vi "Build descriptor.vi"(11 "Builder in":refnum<class "Builder.lvclass">) -> (3 "Builder out":refnum<class "Builder.lvclass">)   [LabVIEW 2025, in "App-Builder Library.lvlib" / "Builder.lvclass"]
uses:
  Builder.lvclass
  Builder.lvclass/Builder.ctl
  App descriptions.ctl
  Build Type.ctl
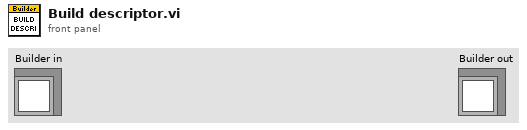
[diagram p1: front panel]
types:
  T1 = typedef "App-Builder Library.lvlib/Builder.lvclass/Build specification.ctl" = cluster{"target name":string, "Build specification":string, "Project Path":path, "Build Object type":T2}
  T2 = typedef "App-Builder Library.lvlib/Builder.lvclass/Build object type.ctl" = enum16{"EXE", "RT EXE", "Deployable Packed"}
  T3 = typedef "App-Builder Library.lvlib/Builder.lvclass/App descriptions.ctl" = cluster{"App Name":string, "Build Type":T4, "Current Version":string, "Next Version":string, "Check":bool}
  T4 = typedef "App-Builder Library.lvlib/Builder.lvclass/Build Type.ctl" = enum16{"Major", "Minor", "Fix", "Build"}
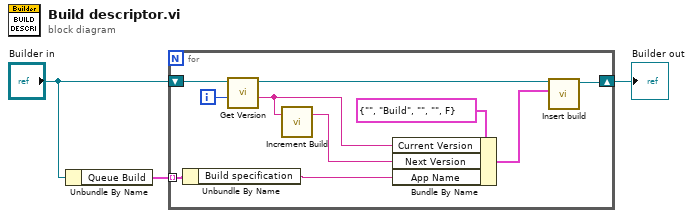
[diagram p0: block diagram]
diagram:
  n1 = Unbundle By Name("Builder in") -> ("Queue Build"=w1:T1[])
  n2 = for {
    tunnel: w1 -> [w5] mode=indexing
    shift-right: [w10] -> w2
    shift-left: "Builder in" -> [w13]
    i -> [w7]
    n3 = Unbundle By Name(w5) -> ("Build specification"=w4:string)
    n4 = call-dynamic "Get Version.vi"("index"=w7, "Builder in"=w13) -> ("Build Version (String)"=w11:string, "Builder out"=w8:refnum<class "Builder.lvclass">)  [unwired: 6 in, 2 out]
    n5 = call "Increment Build.vi"("Current Version"=w11) -> ("next version"=w12:string)  [unwired: 1 in]
    n6 = Bundle By Name(cluster=T3 {"App Name"="", "Build Type"=enum."Build", "Current Version"="", "Next Version"="", "Check"=FALSE} ("Applications"), "Current Version"=w11, "Next Version"=w12, "App Name"=w4) -> (w9:T3)
    n7 = call "Insert build.vi"("Application"=w9, "Builder in"=w8) -> ("Builder out"=w10:refnum<class "Builder.lvclass">)  [unwired: 9 in]
  }
  "Builder out" <- w2
